vi "write U8s.vi"(9 "values":u8[](array[numeric]), 10 "indices":i32[](array[numeric]), 11 "data table in":T1) -> (3 "data table out":T1)   [LabVIEW 2013, in "tag bus.lvlib" / "data table.lvlib"]
doc: "Writes a set of values to the data table. Requires an index for every value."
uses:
  data table.lvlib
  data table.ctl
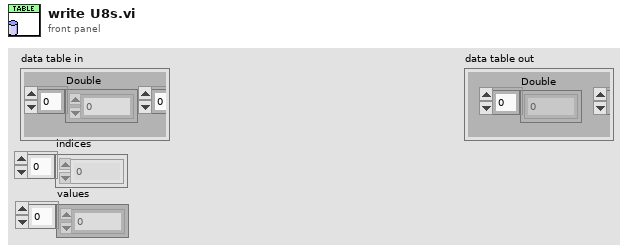
[diagram p1: front panel]
types:
  T1 = typedef "tag bus.lvlib/data table.lvlib/data table.ctl" = cluster{"Double":dbl[], "Single":sgl[], "I64":i64[], "I32":i32[], "I16":i16[], "I8":i8[], "U64":u64[], "U32":u32[], "U16":u16[], "U8":u8[], "Boolean":bool[], "String":string[], "Array of Double":cluster{"DBL Array":dbl[]}[], "Array of Single":cluster{"SGL Array":sgl[]}[], "Array of I64":cluster{"I64 Array":i64[]}[], "Array of I32":cluster{"I32 Array":i32[]}[], "Array of I16":cluster{"I16 Array":i16[]}[], "Array of I8":cluster{"I8 Array":i8[]}[], "Array of U64":cluster{"U64 Array":u64[]}[], "Array of U32":cluster{"U32 Array":u32[]}[], "Array of U16":cluster{"U16 Array":u16[]}[], "Array of U8":cluster{"U8 Array":u8[]}[], "Array of Boolean":cluster{"Boolean Array":bool[]}[], "Array of String":cluster{"String Array":string[]}[]}
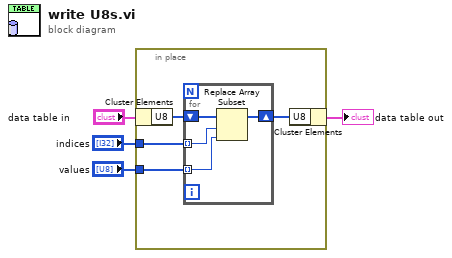
[diagram p0: block diagram]
diagram:
  n1 = in-place {
    in-place-border: "indices" -> [w6]
    in-place-border: "values" -> [w5]
    n2 = in-place-cluster #1("data table in") -> ("U8"=w8:u8[])
    n3 = for {
      tunnel: w6 -> [w12] mode=indexing
      tunnel: w5 -> [w11] mode=indexing
      shift-right: [w9] -> w7
      shift-left: w8 -> [w10]
      n4 = Replace Array Subset(array=w10, new element=w11, index=w12) -> (w9:u8[])
    }
    n5 = in-place-cluster #1("U8"=w7) -> (→"data table out":T1)
  }
